vi "getRepeatabilityError.vi"(9 "检定次数":i32=1, 10 "压力点个数":i32, 11 "温度点一维数组数据":dbl[](array[numeric])) -> (3 "标准偏差":dbl)   [LabVIEW 2017]
panel:
  out "数组 2":dbl[][](array[numeric])
  out "数组":dbl[][](array[numeric])
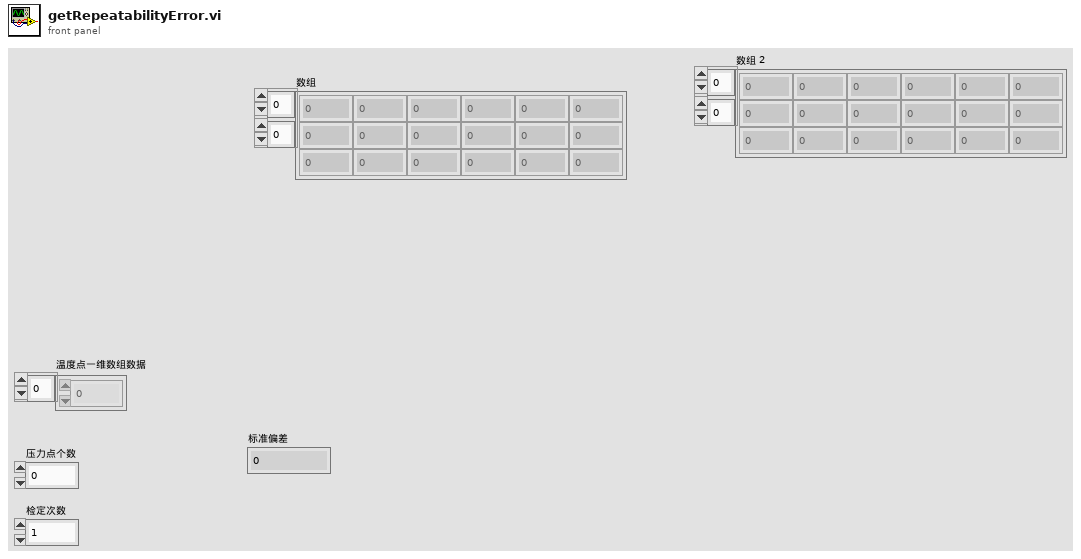
[diagram p1: front panel]
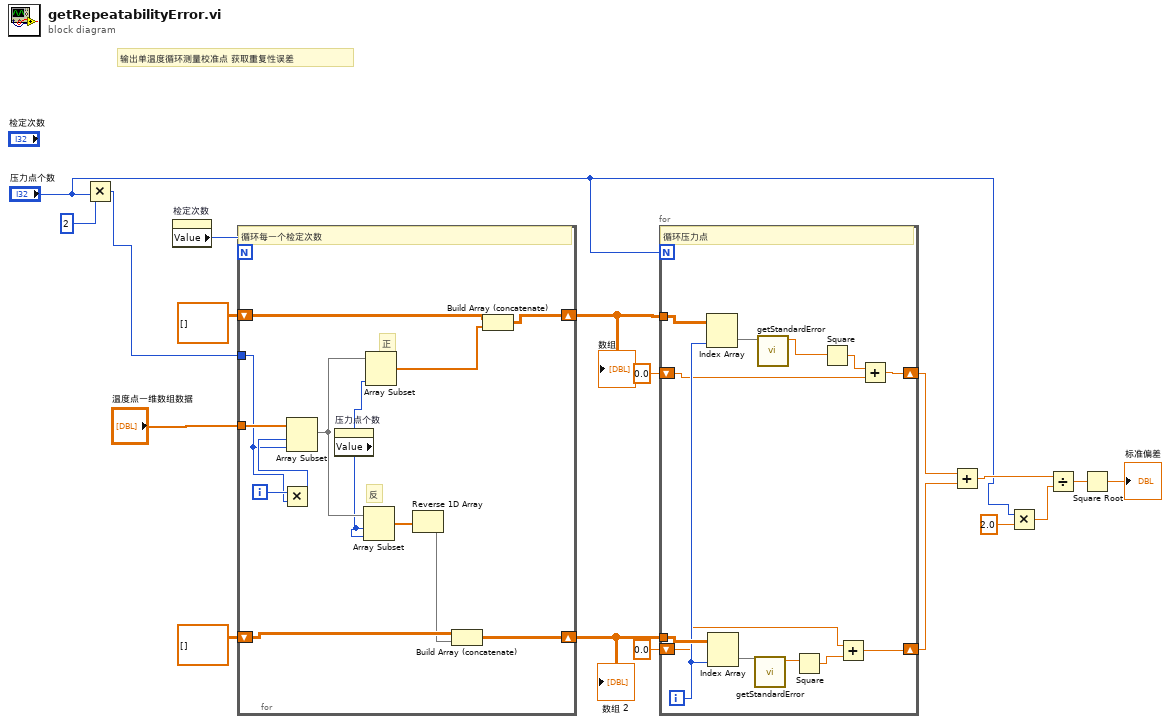
[diagram p0: block diagram]
diagram:
  # "输出单温度循环测量校准点 获取重复性误差"
  n1 = Multiply(x=2, y="压力点个数") -> (x*y=w16:i32)
  n2 = property on="检定次数" class="DigNum (严格)"() -> ("Value"=w17:i32)  [unwired: 2 in, 2 out]
  n3 = for {
    N: w17 -> [_]
    tunnel: w16 -> [w28]
    shift-right: [w22] -> w12
    shift-left: dbl[][] [] -> [w24]
    shift-right: [w19] -> w11
    shift-left: dbl[][] [] -> [w21]
    tunnel: "温度点一维数组数据" -> [w30]
    i -> [w31]
    # "正"
    # "反"
    # "循环每一个检定次数"
    n4 = Multiply(x=w31, y=w28) -> (x*y=w29:i32)
    n5 = Array Subset(array=w30, index=w29, length=w28) -> (w27:dbl[])
    n6 = property on="压力点个数" class="DigNum (严格)"() -> ("Value"=w26:i32)  [unwired: 2 in, 2 out]
    n7 = Array Subset(array=w27, index=w26, length=w26) -> (w25:dbl[])
    n8 = Array Subset(array=w27, length=w26) -> (w23:dbl[])  [unwired: 1 in]
    n9 = Reverse 1D Array(array=w25) -> (reversed array=w20:dbl[])
    n10 = Build Array (concatenate)(w21, w20) -> (w19:dbl[][])
    n11 = Build Array (concatenate)(w24, w23) -> (w22:dbl[][])
  }
  "数组" <- w12
  "数组 2" <- w11
  n12 = for {
    N: "压力点个数" -> [_]
    tunnel: w12 -> [w44]
    tunnel: w11 -> [w43]
    shift-right: [w37] -> w8
    shift-left: 0.0 -> [w36]
    shift-right: [w33] -> w7
    shift-left: 0.0 -> [w32]
    i -> [w42]
    # "循环压力点"
    n13 = Index Array(array=w44, index (col)=w42) -> (element=w41:dbl[])  [unwired: 1 in]
    n14 = Index Array(array=w43, index (col)=w42) -> (element=w40:dbl[])  [unwired: 1 in]
    n15 = call "getStandardError.vi"("一维数组"=w40) -> ("标准差"=w35:dbl)  [unwired: 10 in]
    n16 = call "getStandardError.vi"("一维数组"=w41) -> ("标准差"=w39:dbl)  [unwired: 10 in]
    n17 = Square(x=w35) -> (x^2=w34:dbl)
    n18 = Square(x=w39) -> (x^2=w38:dbl)
    n19 = Add(x=w32, y=w34) -> (x+y=w33:dbl)
    n20 = Add(x=w38, y=w36) -> (x+y=w37:dbl)
  }
  n21 = Add(x=w8, y=w7) -> (x+y=w6:dbl)
  n22 = Multiply(x="压力点个数", y=2.0) -> (x*y=w3:dbl)
  n23 = Divide(x=w6, y=w3) -> (x/y=w2:dbl)
  n24 = Square Root(x=w2) -> (sqrt(x)=→"标准偏差":dbl)
